vi "Draw Scale Line.vi"(9 "BG Image Property In":T1={"Radius"=[], "Plot Area Bounds"={"Left"=0, "Top"=0, "Right"=0, "Bottom"=0}, "Center position"={"X"=0, "Y"=0}, "Flip?"=FALSE, "Major Gird Color"=10066176, "Minor Gird Color"=5000192}, 11 "Picture In":picture) -> (1 "BG Image Property Out":T1={"Radius"=[], "Plot Area Bounds"={"Left"=0, "Top"=0, "Right"=0, "Bottom"=0}, "Center position"={"X"=0, "Y"=0}, "Flip?"=FALSE, "Major Gird Color"=10066176, "Minor Gird Color"=5000192}, 3 "Picture Out":picture)   [LabVIEW 2017, in "2D Compass.lvclass"]
uses:
  <vilib>/Math Plots/2D Math Plots/2D Compass/2D Compass/2D Compass.lvclass
  <vilib>/Math Plots/2D Math Plots/2D Compass/2D Compass/Typedef/BG Image Property.ctl
  <vilib>/Utility/miscctls.llb/LVRectTypeDef.ctl
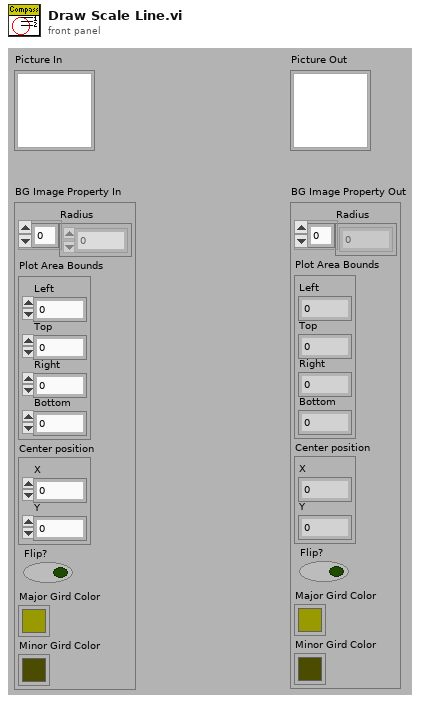
[diagram p1: front panel]
types:
  T1 = typedef "2D Compass.lvclass/BG Image Property.ctl" = cluster{"Radius":i16[], "Plot Area Bounds":T2, "Center position":cluster{"X":i16, "Y":i16}, "Flip?":bool, "Major Gird Color":u32, "Minor Gird Color":u32}
  T2 = typedef "LVRectTypeDef.ctl" = cluster{"Left":i16, "Top":i16, "Right":i16, "Bottom":i16}
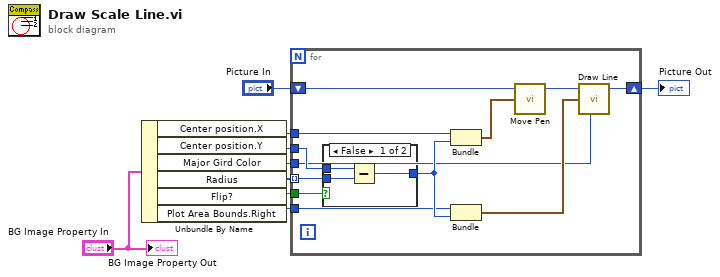
[diagram p0: block diagram]
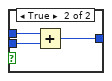
[diagram p2: hidden frame]
diagram:
  n1 = Unbundle By Name("BG Image Property In") -> ("Center position.X"=w9:i16, "Center position.Y"=w8:i16, "Major Gird Color"=w7:u32, "Radius"=w6:i16[], "Flip?"=w3:bool, "Plot Area Bounds.Right"=w2:i16)
  n2 = for {
    shift-right: [w19] -> w4
    shift-left: "Picture In" -> [w21]
    tunnel: w9 -> [w11]
    tunnel: w8 -> [w18]
    tunnel: w7 -> [w14]
    tunnel: w6 -> [w13] mode=indexing
    tunnel: w3 -> [w12]
    tunnel: w2 -> [w10]
    n3 = case shown="False" w12 {
      tunnel: w18 -> [w24 w26]
      tunnel: [w23 w25] -> w17
      tunnel: w13 -> [w22 w27]
      frame False {
        n4 = Subtract(x=w24, y=w22) -> (x-y=w23:i16)
      }
      frame True {
        n5 = Add(x=w26, y=w27) -> (x+y=w25:i16)
      }
    }
    n6 = Bundle("X"=w11, w17) -> (w15:cluster{"X":i16, i16})  [unwired: 1 out]
    n7 = Bundle("Right"=w10, w17) -> (w16:cluster{"Right":i16, i16})  [unwired: 1 out]
    n8 = call <vilib>:"Move Pen.vi"("new position"=w15, "picture"=w21) -> ("new picture"=w20:picture)  [unwired: 1 in, 2 out]
    n9 = call <vilib>:"Draw Line.vi"("picture"=w20, "end point"=w16, "color(black)"=w14) -> ("new picture"=w19:picture)  [unwired: 2 in, 4 out]
  }
  "Picture Out" <- w4
  "BG Image Property Out" <- "BG Image Property In"
